vi "NI VeriStand - Get Parameters List.vi"(7 "Target":string, 8 "error in (no error)":errorcluster, 11 "ModelManager in":T1) -> (0 "error out":errorcluster, 2 "Parameters":string[](array[string]), 3 "ModelManager out":T1)   [LabVIEW 2020, in "NI_VS ModelManager ExecutionAPI.lvlib"]
doc: "Returns a list of all the parameters for all models present on the target."
uses:
  <vilib>/NI VeriStand/Execution/ModelManager/NI_VS ModelManager ExecutionAPI.lvlib
  <vilib>/NI VeriStand/Execution/ModelManager/ModelManagerAPI.ctl
  NationalInstruments.VeriStand.ClientAPI
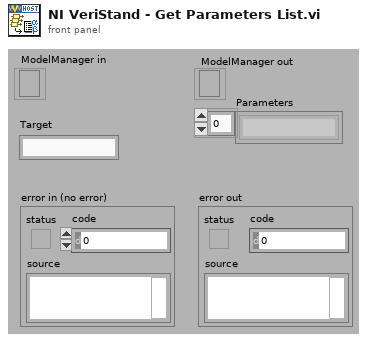
[diagram p1: front panel]
types:
  T1 = typedef "NI_VS ModelManager ExecutionAPI.lvlib/ModelManagerAPI.ctl" = refnum<k24>
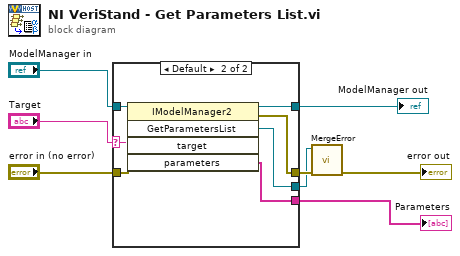
[diagram p0: block diagram]
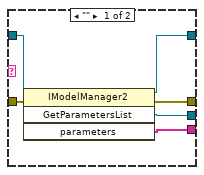
[diagram p2: hidden frame]
diagram:
  n1 = case shown="Default" "Target" {
    selector: "Target" -> [_ w16]
    tunnel: "ModelManager in" -> [w14 w21]
    tunnel: [w13 w20] -> w7
    tunnel: [w12 w19] -> w6
    tunnel: [w11 w18] -> w5
    tunnel: "error in (no error)" -> [w10 w17]
    tunnel: [w9 w15] -> w2
    frame "" {
      n2 = invoke class="IModelManager2" method="GetParametersList"(reference=w14, error in=w10) -> (reference out=w13:T1, error out=w12:errorcluster, "GetParametersList"=w11:refnum<k24>, "parameters"=w9:string[])  [unwired: 2 in]
    }
    frame Default {
      n3 = invoke class="IModelManager2" method="GetParametersList"(reference=w21, error in=w17, "target"=w16) -> (reference out=w20:T1, error out=w19:errorcluster, "GetParametersList"=w18:refnum<k24>, "parameters"=w15:string[])  [unwired: 2 in, 1 out]
    }
  }
  "ModelManager out" <- w7
  "Parameters" <- w2
  n4 = call <vilib>:"MergeError.vi"("error in (no error)"=w6, "Error"=w5) -> ("error out"=→"error out":errorcluster)  [unwired: 9 out]
